vi "FindDaysBackMinNotLog.vi"(10 "Cluster":cluster{i32[], timestamp[]}) -> (1 "Index":i32, 2 "Error":dbl, 3 "Growth":dbl)   [LabVIEW 2017]
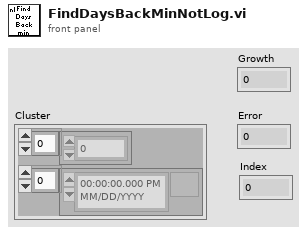
[diagram p1: front panel]
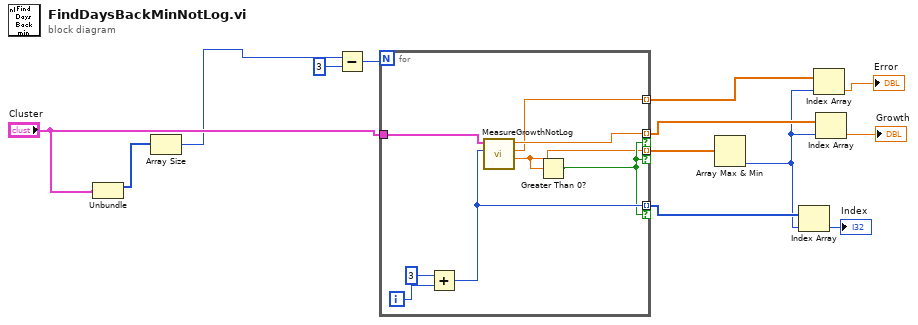
[diagram p0: block diagram]
diagram:
  n1 = Unbundle("Cluster") -> (w7:i32[])  [unwired: 1 out]
  n2 = Array Size(array=w7) -> (size(s)=w6:i32)
  n3 = Subtract(x=w6, y=3) -> (x-y=w10:i32)
  n4 = for {
    N: w10 -> [_]
    tunnel: "Cluster" -> [w17]
    tunnel: [w18] -> w12 mode=indexing if=w16
    tunnel: [w15] -> w11 mode=indexing if=w16
    tunnel: [w19] -> w5 mode=indexing if=w16
    tunnel: [w14] -> w3 mode=indexing
    i -> [w21]
    n5 = Add(x=3, y=w21) -> (x+y=w19:i32)
    n6 = call "MeasureGrowthNotLog.vi"("DaysBack"=w19, "Data"=w17) -> ("Interval"=w15:dbl, "PlusMinus"=w14:dbl, "Growth"=w18:dbl)  [unwired: 3 in, 4 out]
    n7 = Greater Than 0?(x=w15) -> (x > 0?=w16:bool)
  }
  n8 = Array Max & Min(array=w11) -> (min index (indices)=w2:i32)  [unwired: 3 out]
  n9 = Index Array(array=w5, index=w2) -> (element=→"Index":i32)
  n10 = Index Array(array=w3, index=w2) -> (element=→"Error":dbl)
  n11 = Index Array(array=w12, index=w2) -> (element=→"Growth":dbl)
